vi "LibXML_GetNodeStrPtr.vi"(8 "error in":errorcluster, 9 "type":enum16{"NOP", "name", "content"}(ring), 10 "node":u32) -> (0 "error out":errorcluster, 3 "string ptr  out":u32)   [LabVIEW 2019, in "Tools.lvlib" / "LibXML.lvlib"]
doc: "Get the string pointer for the node"
uses:
  LibXML.lvlib
  dll/lXMLwrap.dll
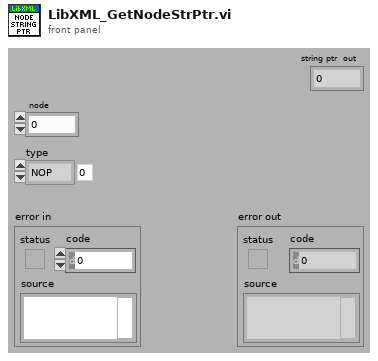
[diagram p1: front panel]
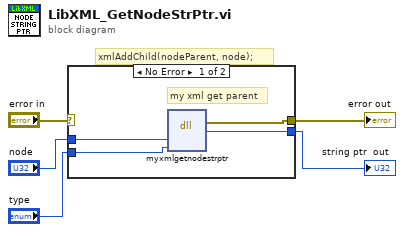
[diagram p0: block diagram]
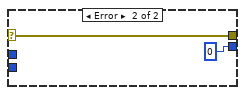
[diagram p2: hidden frame]
diagram:
  # "xmlAddChild(nodeParent, node);"
  n1 = case shown="No Error" "error in" {
    selector: "error in" -> [_ w11]
    tunnel: [w6 w11] -> w4
    tunnel: "node" -> [w9 _]
    tunnel: "type" -> [w8 _]
    tunnel: [w7 u32 0 ("return type")] -> w1
    frame No Error {
      # "my xml get parent"
      n2 = dll-call lib="C:/Projects/_Prywatne/MyCIT/Framework/Tools/XML/LibXML/dll/lXMLwrap.dll" fn="myxmlgetnodestrptr"("node"=w9, "type"=w8) -> (error out=w6:errorcluster, "return type"=w7:u32)  [unwired: 5 in, 1 out]
    }
    frame Error {
    }
  }
  "error out" <- w4
  "string ptr  out" <- w1
